vi "micsTest.vi"() -> ()   [LabVIEW 2017]
uses:
  <vilib>/express/express analysis/Spectral/Block/exnSpectralBlock spectral measurements RMS poly.vi
  <vilib>/express/express analysis/Spectral/Block/exnSpectralBlock spectral measurements RMS DDT.vi
  <vilib>/express/express analysis/Spectral/XNode/ExpressSpectralMeasurementsBlockNode.xnode
panel:
  out "Waveform Graph":dynamicdata(graph)
  out "non filtered":dynamicdata(graph) caption="data"
  out "filtered":dynamicdata(graph) caption="data"
  in  "stop (F)":bool
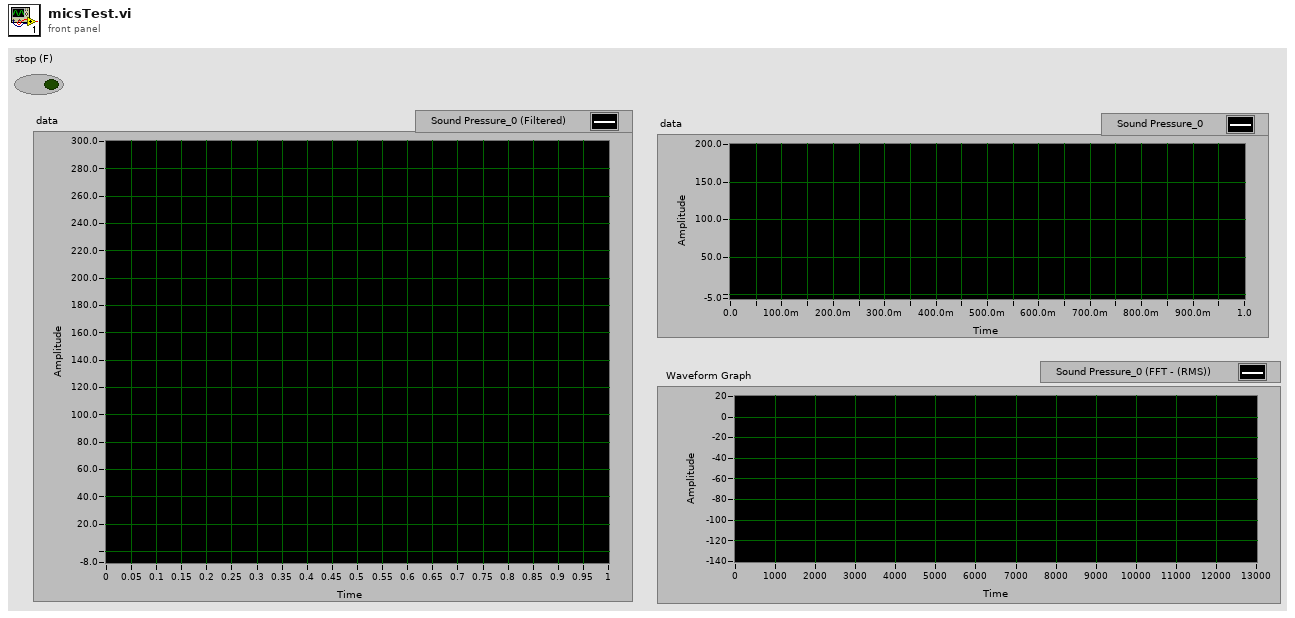
[diagram p1: front panel]
types:
  T1 = cluster{"averaging mode":u16, "weighting mode":u16, "number of averages":u32}
  T2 = cluster{"dB On (F)":bool, "unwrap phase (F)":bool, "convert to degree (F)":bool}
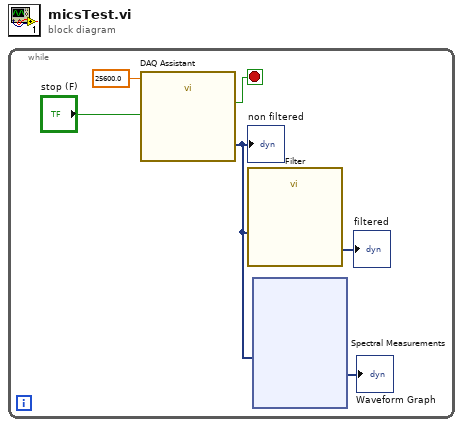
[diagram p0: block diagram]
diagram:
  n1 = while {
    stop <- w5 stop-if-true
    n2 = call "DAQ Assistant"("rate"=25600.0, "stop (F)"="stop (F)") -> ("data"=w2:dynamicdata, "stopped"=w5:bool)  [unwired: 14 in, 2 out]
    "non filtered" <- w2
    n3 = call "Filter"("Signal"=w2) -> ("Filtered Signal"=→"filtered":dynamicdata)  [unwired: 9 in, 1 out]
    n4 = xnode "Spectral Measurements"("Signals"=w2) -> ("FFT - (RMS)"=→"Waveform Graph":dynamicdata)  [unwired: 1 in, 2 out]
  }
